vi "GetDataForExcel.vi"(8 "error in (no error)":errorcluster, 9 "ID":string, 10 "ReportSelection":u16, 11 "closing behavior (leave open)":T1(ring)) -> (0 "error out":errorcluster, 1 "ExcelError":bool, 3 "ReportPath":path)   [LabVIEW 2013, in "main.lvlib"]
uses:
  main.lvlib
  <userlib>/_OpenG.lib/file/file.llb/File Exists - Scalar__ogtk.vi
  <vilib>/regexp/Match Regular Expression.xnode
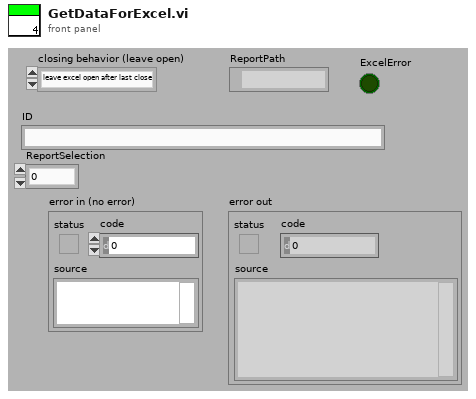
[diagram p1: front panel]
types:
  T1 = enum16{"leave excel open after last close", "close only if opened by LabVIEW", "close excel after last close"}
  T2 = cluster{"Dicom Values":string[][], "Date":string, "Palpation":string[], "Personal Info":string[], "Hospital":string[], "Path":path}
  T3 = cluster{"Palpation":string[], "Personal Info":string[], "Hospital":string[]}
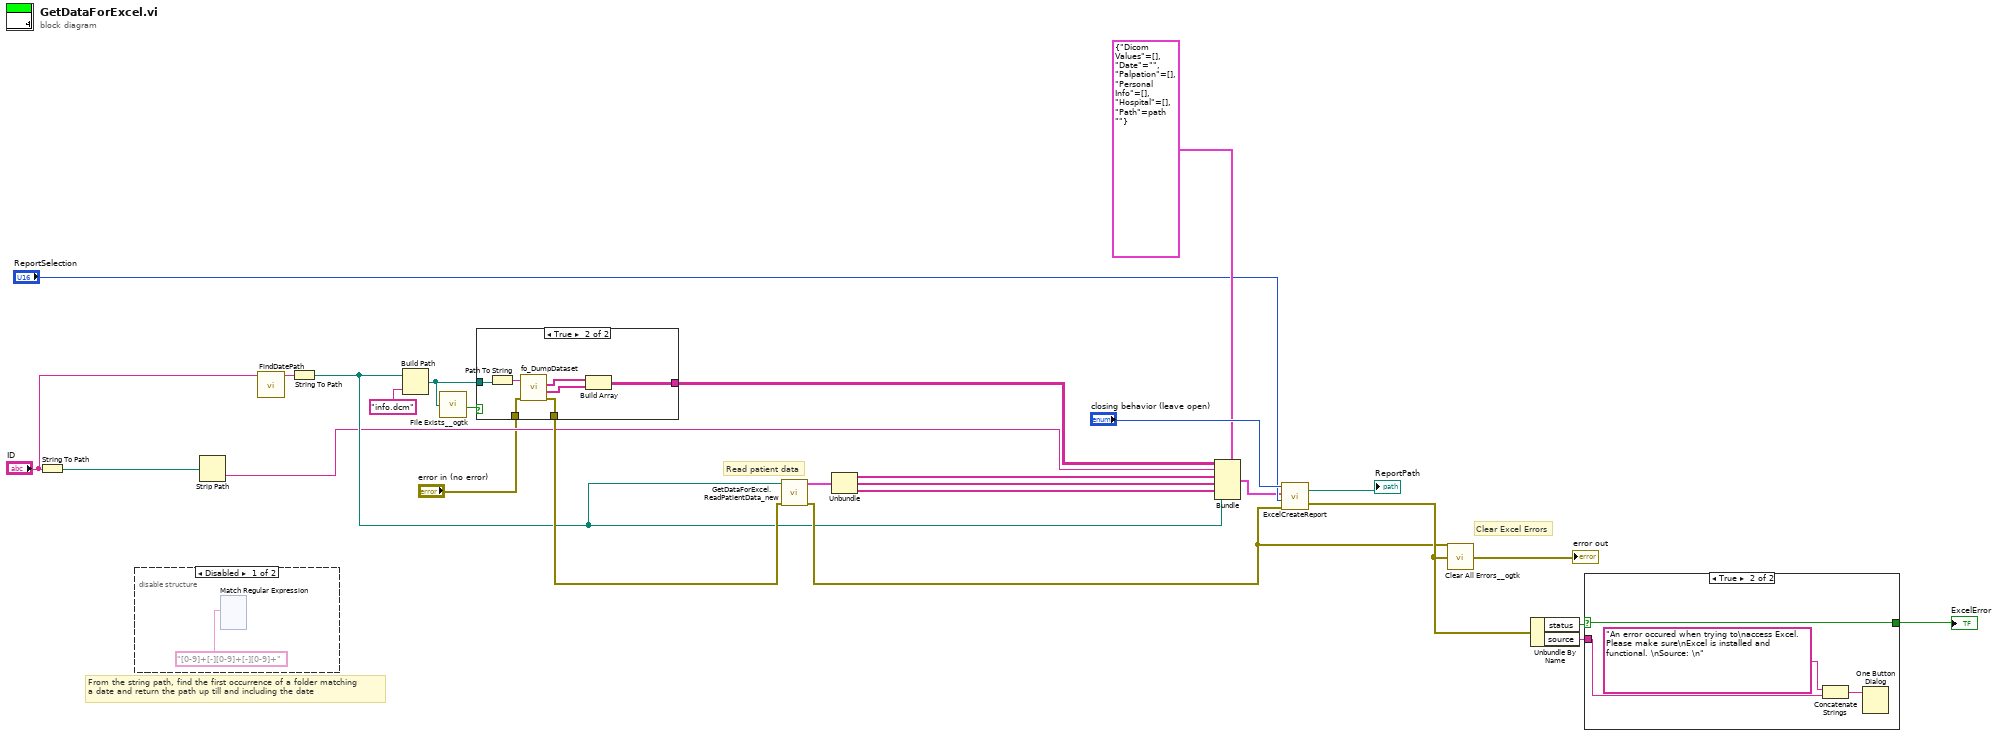
[diagram p0: block diagram]
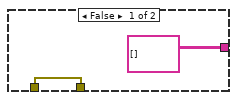
[diagram p3: hidden frame]
diagram:
  # "From the string path, find the first occurrence of a folder matching\na date and return the path up till and including the date"
  # "Read patient data"
  # "Clear Excel Errors"
  n1 = String To Path(string="ID") -> (path=w2:path)
  n2 = disable-structure shown="Disabled" {
    frame Disabled {
      n3 = xnode "Match Regular Expression"("regular expression"="[0-9]+[-][0-9]+[-][0-9]+") -> ()  [unwired: 5 in, 5 out]
    }
    frame Enabled {
    }
  }
  n4 = Strip Path(path=w2) -> (name=w4:string)  [unwired: 1 out]
  n5 = call "FindDatePath.vi"("Message Value"="ID") -> ("String"=w6:string)  [unwired: 10 in]
  n6 = String To Path(string=w6) -> (path=w5:path)
  n7 = Build Path(base path=w5, name or relative path="info.dcm") -> (appended path=w19:path)
  n8 = call-poly <userlib>:"File Exists__ogtk.vi"("file path"=w19) -> ("exists"=w18:bool)  [unwired: 6 in, 1 out]
  n9 = case shown="True" w18 {
    tunnel: [string[][] [] w147] -> w20
    tunnel: w19 -> [_ w146]
    tunnel: "error in (no error)" -> [w139 w144]
    tunnel: [w139 w143] -> w8
    frame False {
    }
    frame True {
      n10 = Path To String(path=w146) -> (string=w145:string)
      n11 = call "fo_DumpDataset.vi"("error in (no error)"=w144, "file"=w145) -> ("error out"=w143:errorcluster, "items"=w141:string[], "keywords"=w142:string[])  [unwired: 6 in, 1 out]
      n12 = Build Array(w142, w141) -> (w147:string[][])
    }
  }
  n13 = call "GetDataForExcel.ReadPatientData_new.vi"("error in"=w8, "Path"=w5) -> ("error out"=w7:errorcluster, "output cluster"=w17:T3)  [unwired: 8 in]
  n14 = Unbundle(w17) -> ("Palpation"=w13:string[], "Personal Info"=w11:string[], "Hospital"=w10:string[])
  n15 = Bundle(cluster=T2 {"Dicom Values"=[], "Date"="", "Palpation"=[], "Personal Info"=[], "Hospital"=[], "Path"=path ""}, "Dicom Values"=w20, "Date"=w4, "Palpation"=w13, "Personal Info"=w11, "Hospital"=w10, "Path"=w5) -> (w9:T2)
  n16 = call "ExcelCreateReport.vi"("error in (no error)"=w7, "ReportSelection"="ReportSelection", "Input"=w9, "closing behavior"="closing behavior (leave open)") -> ("error out"=w16:errorcluster, "ReportPath"=→"ReportPath":path)
  n17 = call <userlib>:"Clear All Errors__ogtk.vi"("Upsteam Error (optional)"=w7, "Error In"=w16) -> ("Error Out"=→"error out":errorcluster)  [unwired: 2 in]
  n18 = Unbundle By Name(w16) -> ("status"=w23:bool, "source"=w15:string)
  n19 = case shown="True" w23 {
    selector: w23 -> [w148 w152]
    tunnel: [w148 w152] -> w22
    tunnel: w15 -> [_ w150]
    frame False {
    }
    frame True {
      n20 = Concatenate Strings("An error occured when trying to\naccess Excel. Please make sure\nExcel is installed and functional. \nSource: \n" ("message"), w150) -> (w149:string)
      n21 = One Button Dialog(message=w149) -> ()  [unwired: 1 in, 1 out]
    }
  }
  "ExcelError" <- w22
